vi "UpdateMovingCursor.vi"(8 "Coords":T1, 9 "CtlRef":refnum<vi>) -> ()   [LabVIEW 2013, in "main.lvlib"]
uses:
  main.lvlib
  <vilib>/Utility/miscctls.llb/LVPoint32TypeDef.ctl
  Controls/Enum Variables.ctl
  <vilib>/Analysis/6fits.llb/Curve Fitting Criteria.ctl
  <vilib>/Analysis/NI_AALPro.lvlib
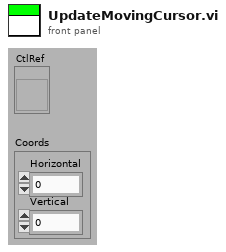
[diagram p1: front panel]
types:
  T1 = typedef "LVPoint32TypeDef.ctl" = cluster{"Horizontal":i32, "Vertical":i32}
  T2 = typedef "main.lvlib/Enum Variables.ctl" = enum16{"SetAcqFilter", "GetAcqFilter", "Set Filter", "Get Filter", "Set Height", "Get Height", "Set Recorded Height", "Get Recorded Height", "Set Blue Pressure", "Get Blue Pressure", "Set Red Pressure", "Get Red Pressure", "Init", "Reset Pressure", "Set Red Cursors", "Get Red Cursors", "Set Blue Cursors", "Get Blue Cursors", "Set Language", "Get Language", "Set Active Graphs", "Get ActiveGraphs", "Set Method", "Get Method", "Set Encryption", "Get Encryption", "Set ExcelVersion", "Get ExcelVersion", "Set DICOM Avail", "Get DICOM Avail", "Set DICOM Encode", "Get DICOM Encode", "Set JournalExport", "Get JournalExport", "Set Sequence", "Get Sequence", "Set DAQ Connected", "Get DAQ Connected", "Set Current Graph", "Get Current Graph", "Set General Settings", "Get Hyphenation", "Set Arm Calc Method", "Get Arm Calc Method", "Set Dicom Tags", "Get Dicom Tags", "Set BT Serial", "Get BT Serial", "Set BT Accepted Serials", "Get BT Accepted Serials", "Get BT License", "Set BT License"}
  T3 = typedef "NI_AALPro.lvlib/Curve Fitting Criteria.ctl" = u16
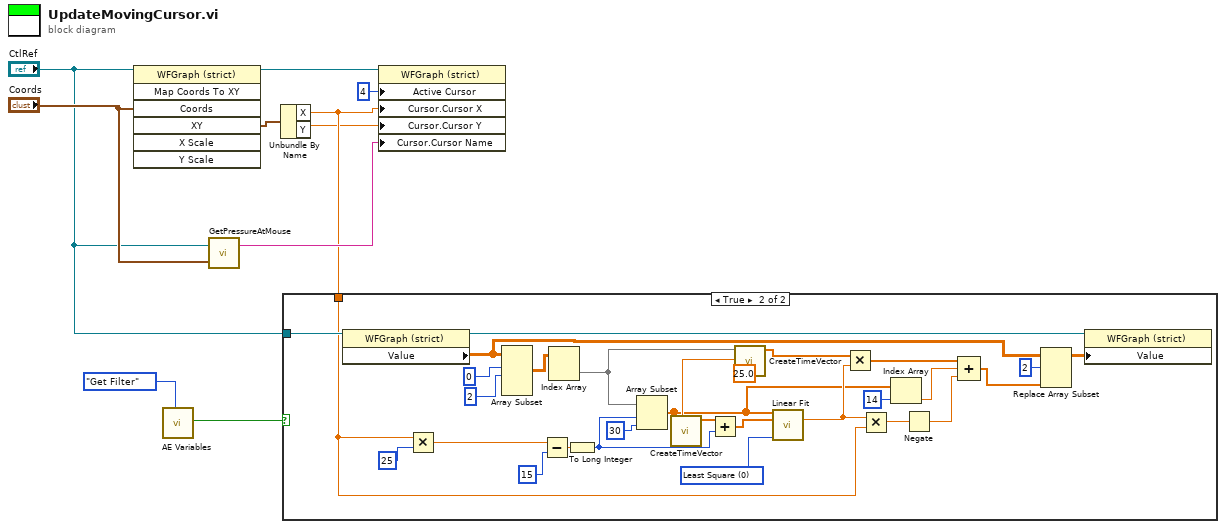
[diagram p0: block diagram]
diagram:
  n1 = invoke class="WFGraph (strict)" method="Map Coords To XY"(reference="CtlRef", "Coords"="Coords") -> (reference out=w7:refnum<vi>, "XY"=w1:cluster{"X":dbl, "Y":dbl})  [unwired: 5 in, 5 out]
  n2 = call "AE Variables.vi"("Action"=Enum_Variables."Get Filter") -> ("BooleanOut"=w3:bool)  [unwired: 11 in, 7 out]
  n3 = call "GetPressureAtMouse.vi"("Coords"="Coords", "GraphRefnum"="CtlRef") -> ("String"=w9:string)  [unwired: 1 out]
  n4 = Unbundle By Name(w1) -> ("X"=w4:dbl, "Y"=w2:dbl)
  n5 = case shown="True" w3 {
    tunnel: "CtlRef" -> [_ w39]
    tunnel: w4 -> [_ w18]
    frame False {
    }
    frame True {
      w28 = 25.0 ("Sampling Frequency")
      w38 = T3 0 items=["Least Square", "Least Absolute Residual", "Bisquare"] ("method")
      n6 = property class="WFGraph (strict)"(reference=w39) -> (reference out=w34:refnum<vi>, "Value"=w14:dbl[][])  [unwired: 1 in, 1 out]
      n7 = Multiply(x=w18, y=25) -> (x*y=w30:dbl)
      n8 = Array Subset(array=w14, index (row)=0 ("index"), length (row)=2 ("length")) -> (w26:dbl[][])  [unwired: 2 in]
      n9 = Subtract(x=w30, y=15 ("length")) -> (x-y=w36:dbl)
      n10 = Index Array(array=w26) -> (element=w35:dbl[])  [unwired: 2 in]
      n11 = To Long Integer(number=w36) -> (32bit integer=w22:i32)
      n12 = Array Subset(array=w35, index=w22, length=30) -> (w21:dbl[])
      n13 = call "CreateTimeVector.vi"("Sampling Frequency"=w28, "Array in"=w21) -> ("Array out"=w33:dbl[])  [unwired: 9 in]
      n14 = Add(x=w33, y=w22) -> (x+y=w32:dbl[])
      n15 = call "CreateTimeVector.vi"("Sampling Frequency"=w28, "Array in"=w35) -> ("Array out"=w29:dbl[])  [unwired: 9 in]
      n16 = call <vilib>:"Linear Fit.vi"("Y"=w21, "X"=w32, "method"=w38) -> ("slope"=w23:dbl)  [unwired: 8 in, 4 out]
      n17 = Multiply(x=w29, y=w23) -> (x*y=w27:dbl[])
      n18 = Multiply(x=w23, y=w18) -> (x*y=w17:dbl)
      n19 = Index Array(array=w21, index=14) -> (element=w15:dbl)
      n20 = Negate(x=w17) -> (-x=w16:dbl)
      n21 = Compound Arithmetic op=ADD(w27, w15, w16) -> (w12:dbl[])
      n22 = Replace Array Subset(array=w14, new element=w12, index (row)=2) -> (w13:dbl[][])  [unwired: 1 in]
      n23 = property class="WFGraph (strict)"(reference=w34, "Value"=w13) -> ()  [unwired: 1 in, 2 out]
    }
  }
  n24 = property class="WFGraph (strict)"(reference=w7, "Active Cursor"=u32 4, "Cursor.Cursor X"=w4, "Cursor.Cursor Y"=w2, "Cursor.Cursor Name"=w9) -> ()  [unwired: 1 in, 2 out]
